vi "MARS_Analysis.vi"() -> ()   [LabVIEW 2015]
uses:
  <vilib>/Analysis/6fits.llb/Curve Fitting Criteria.ctl
  SubVis/MARS_Global_var.vi
  SubVis/Data_Analysis_subvis/MARS_Scan_Data_Analysis_global.vi
  SubVis/Data_Analysis_subvis/ESA_Data_Analysis_Global_VIs.vi
  SubVis/MARS_Scan_Global_var.vi
  <vilib>/Analysis/NI_AALPro.lvlib
panel:
  in  "index":i32=1
  in  "Init std":dbl=1.0 format="%#_13g"
  in  "width":i32=5
  in  "threshold":dbl=10.0 format="%#_13g"
  in  "Discr. Slope":dbl
  in  "Discr. Offset":dbl
  out "Total Counts":i32
  out "Gamma Counts":i32
  out "Neutron Counts":i32
  out "Gamma %":dbl format="%#.2f"
  out "Neutron  %":dbl format="%#.2f"
  in  "Spectrum sel.":bool
  out "Indicator":bool
  in  "Page Selector":enum32{"Free Run Tests", "Scanning Tests"}(radio)
  out "Tab Control":enum32{"Free Run Tests", "Scanning Tests"}(tab)
  in  "Inegral Sel":bool
  in  "Mapping":bool
  in  "Boolean 2":bool
  in  "Spec Selec 2":bool
  out "Spectrum":i32[][](graph)
  out "Int. Graph":i32[][](graph) caption="Intensity Graph"
  out "Scatter":T1(graph) caption="Scatter Plot"
  out "Histogram":i32[][](graph)
  out "FoM":dbl
  out "FoM_1st_min":dbl
  out "FoM_2nd_min":dbl
  out "Channels":i32(listbox) caption="Bckgnd_0.50us-6.00us"
  out "FoM_1st_max":dbl
  out "FoM_2nd_max":dbl
  out "FoM_2":dbl caption="FoM"
  out "Histogram 2":i32[][](graph) caption="Histogram"
  out "Ratio Graph":i32[][](graph) caption="Integral Ratio Graph"
  out "FoM Graph":dbl[][](graph) caption="Optimal FoM"
  in  "Stop Button":bool
  in  "Active Meas.":i32
  out "Meas. Duration (s)":dbl format="%^#.3g"
  out "2nd Integr. (us)":dbl format="%^#.2g"
  out "1st Integr. (us)":dbl format="%^#.2g"
  out "Trigger Level (V)":dbl format="%#.3p"
  in  "Listbox":i32[](listbox) caption="FreeRun_gamma_tests.tdms"
  in  "Read":bool
  out "error out":errorcluster
  # "ADVEOS\nGAEC\nNCSR DEMOKRITOS"
  # "MARS    Neutron Subsystem   Data Analysis"
  # "Neutron-Gamma\nDiscr. Parameters"
  # "Spectrum Statistics"
  # "Measurement Parameters"
  # "%"
  # "%"
  # "Histogram Fit"
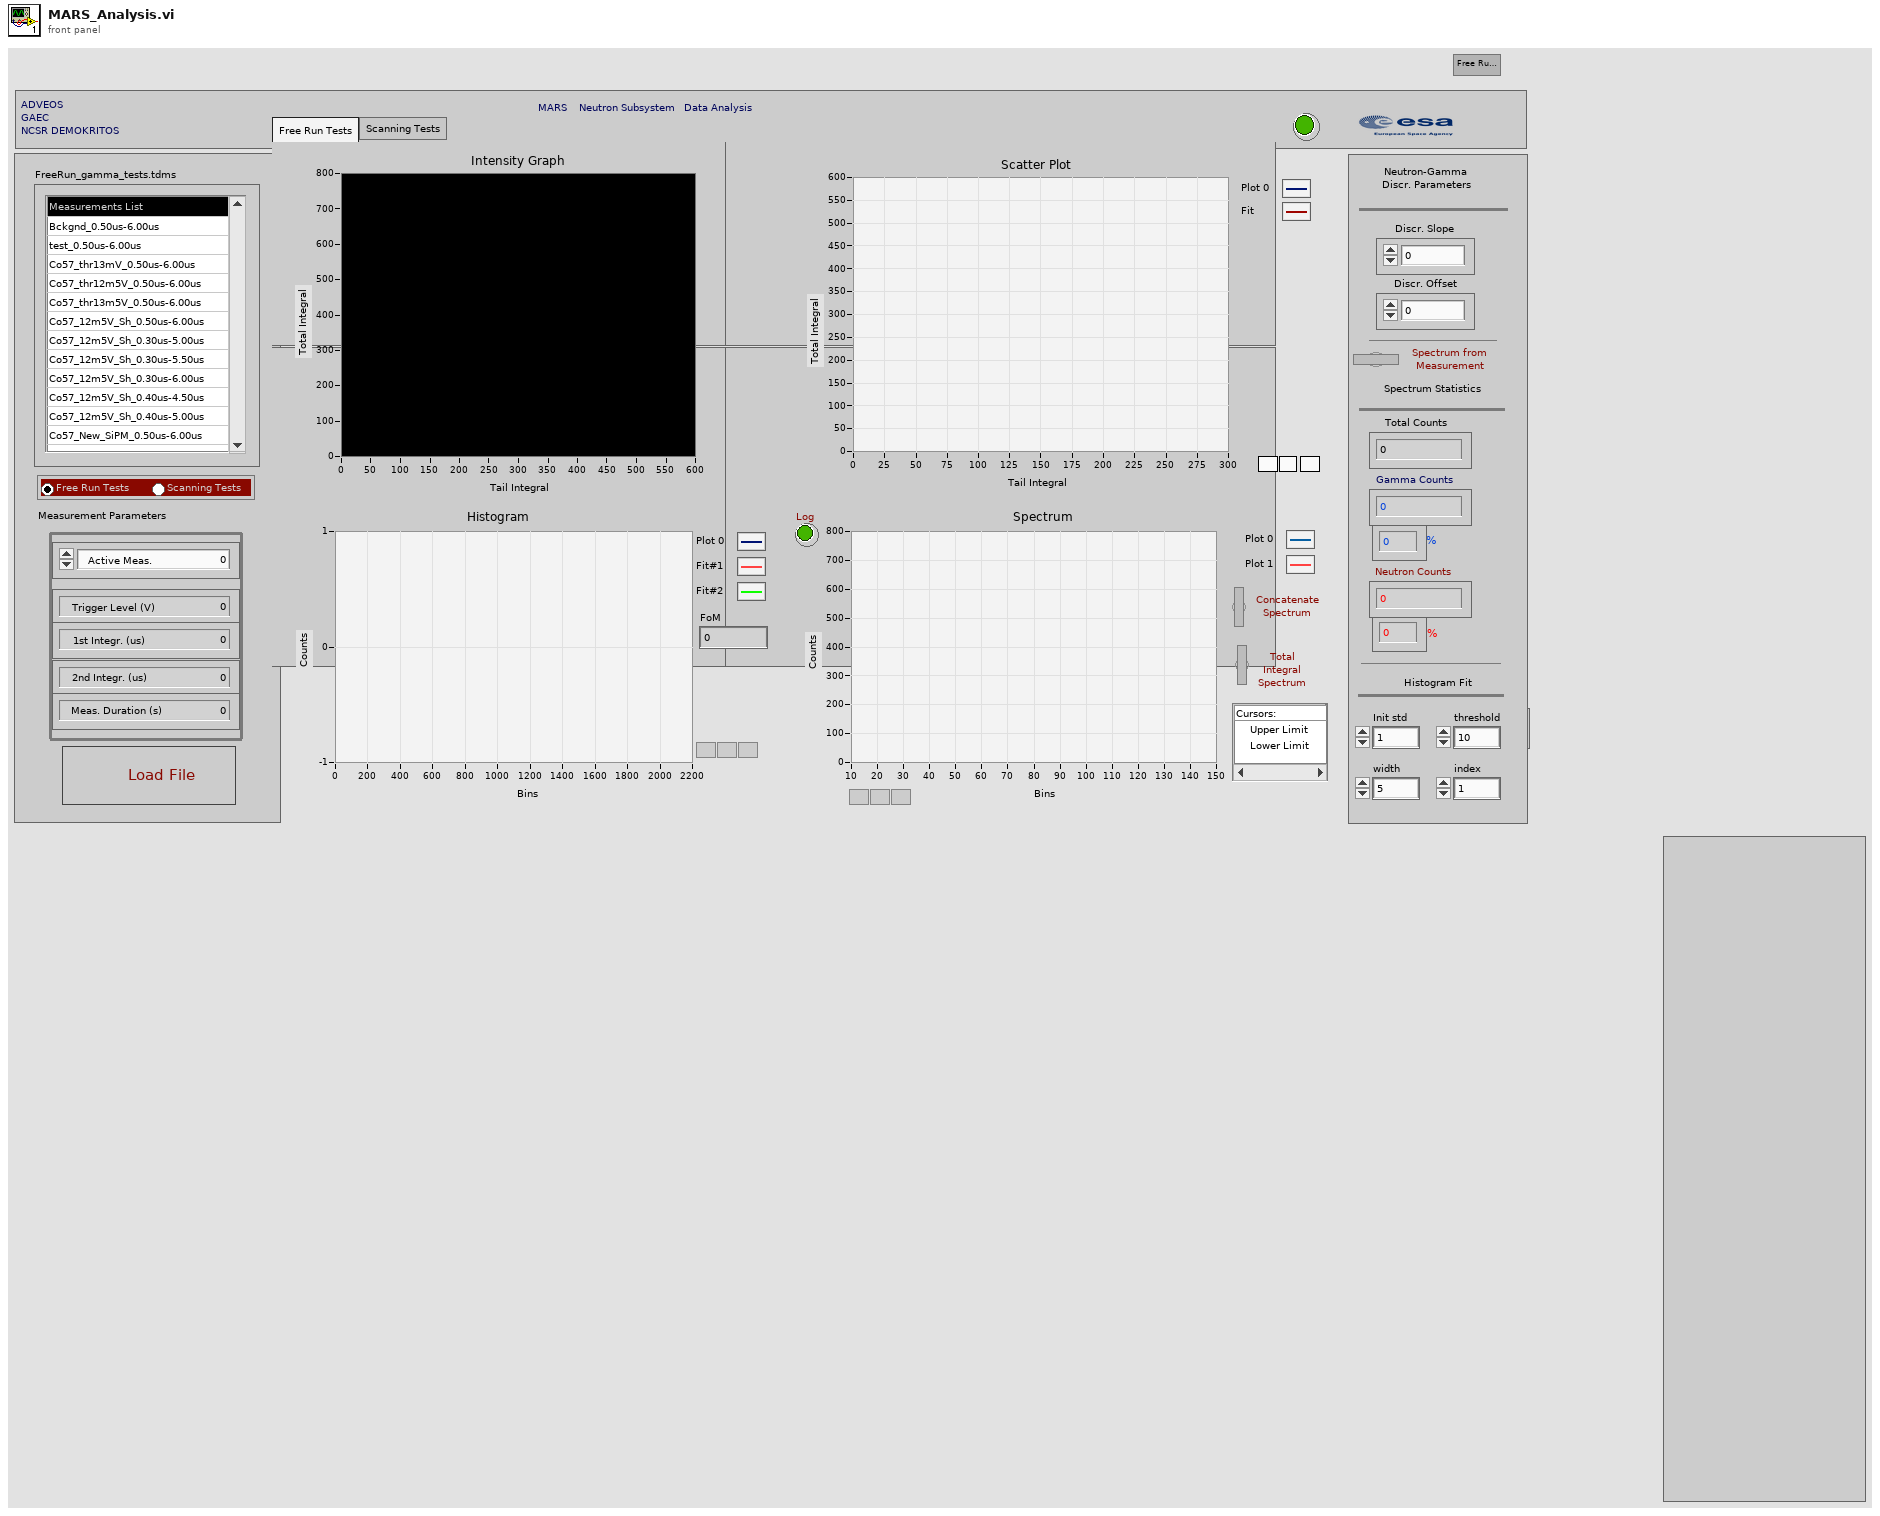
[diagram p1: front panel]
types:
  T1 = cluster{"Tail Integral":i32[], "Total Integral":dbl[]}[]
  T2 = enum16{"open", "open or create", "create or replace", "create", "open (read-only)"}
  T3 = typedef "NI_AALPro.lvlib/Curve Fitting Criteria.ctl" = u16
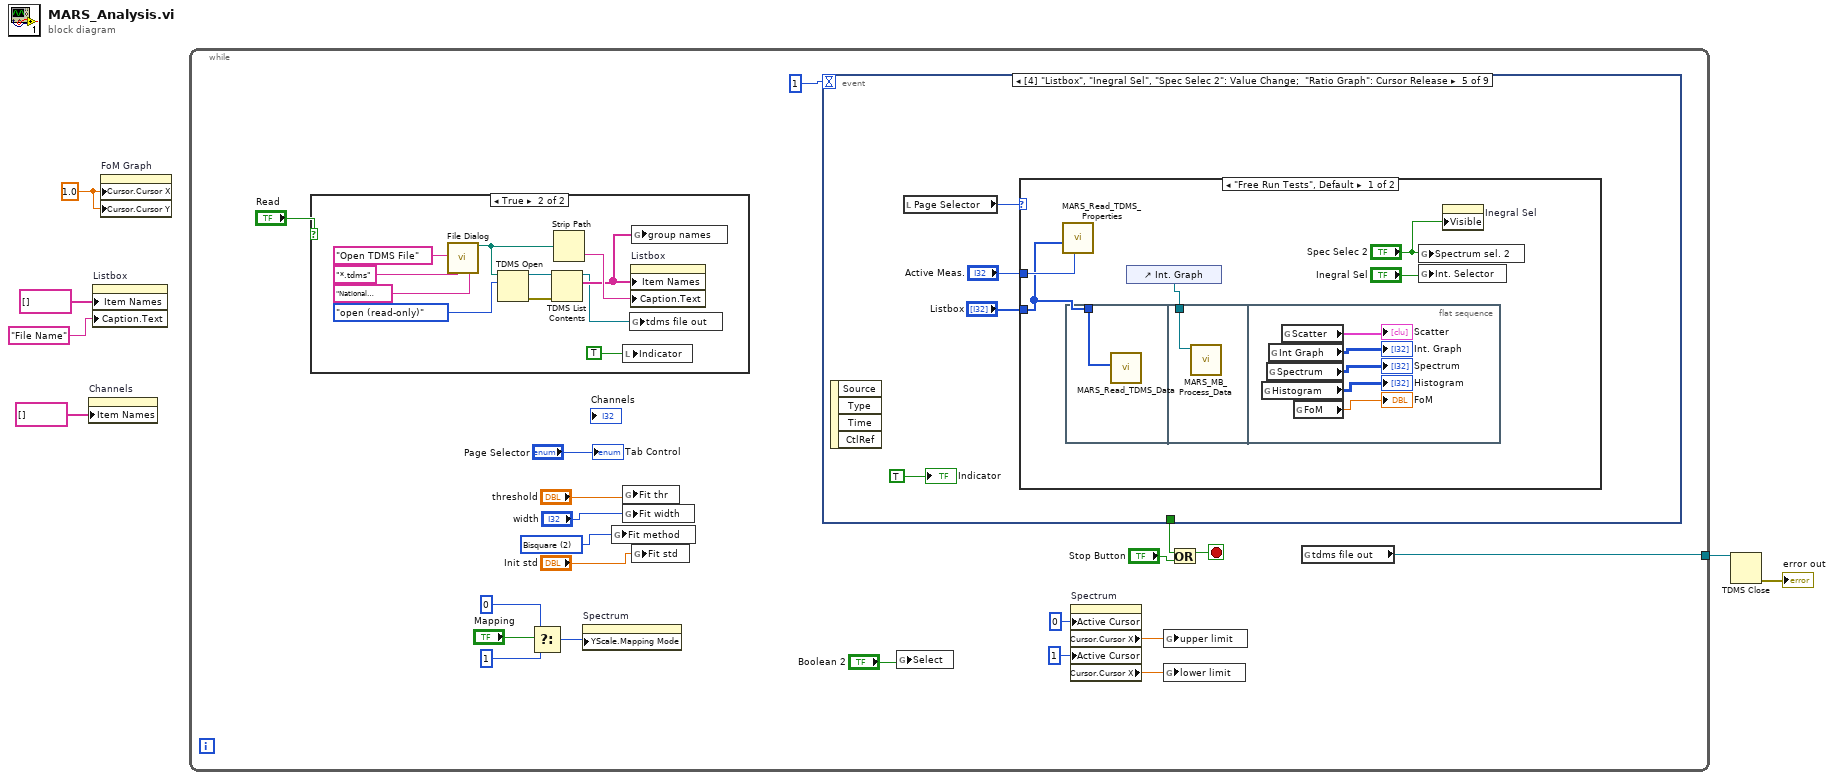
[diagram p0: block diagram]
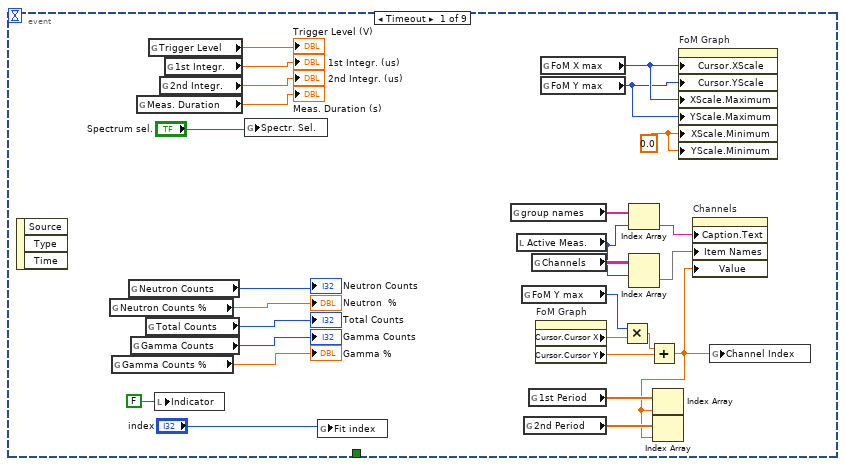
[diagram p3: hidden frame]
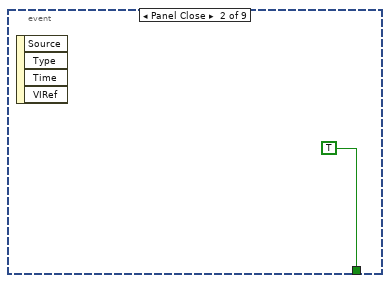
[diagram p4: hidden frame]
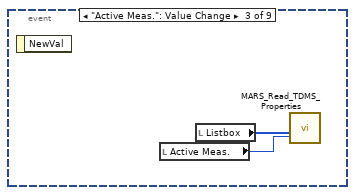
[diagram p5: hidden frame]
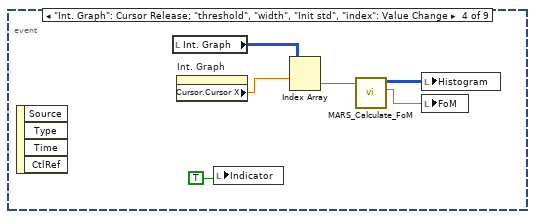
[diagram p6: hidden frame]
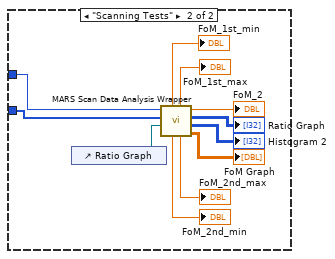
[diagram p7: hidden frame]
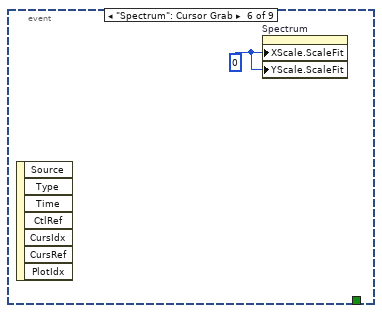
[diagram p8: hidden frame]
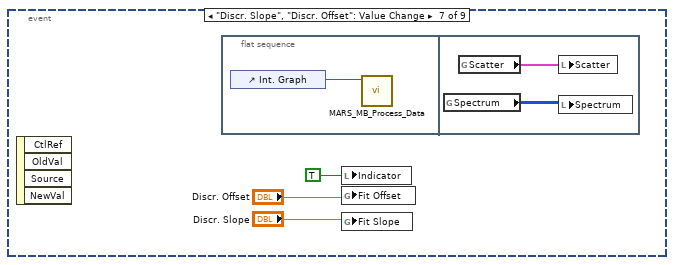
[diagram p9: hidden frame]
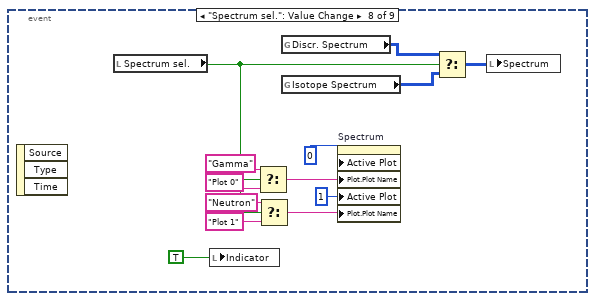
[diagram p10: hidden frame]
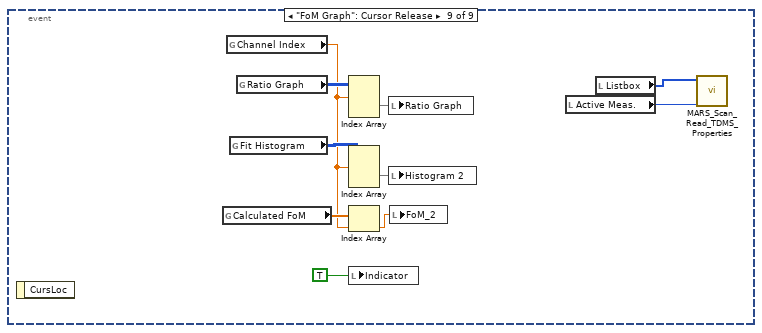
[diagram p11: hidden frame]
diagram:
  w2 = 1.0 ("Cursor.Cursor Position:Cursor X")
  n1 = property on="Channels" class="LstBox (strict)"("Item Names"=string[] []) -> ()  [unwired: 2 in, 2 out]
  n2 = property on="Listbox" class="LstBox (strict)"("Item Names"=string[] [], "Caption.Text"="File Name") -> ()  [unwired: 2 in, 2 out]
  n3 = property on="FoM Graph" class="IntGraph (strict)"("Cursor.Cursor X"=w2, "Cursor.Cursor Y"=w2) -> ()  [unwired: 2 in, 2 out]
  n4 = while {
    tunnel: [w26] -> w6
    stop <- w24 stop-if-true
    w17 = T3 2 items=["Least Square", "Least Absolute Residual", "Bisquare"] ("method")
    n5 = case shown="True" "Read" {
      frame False {
      }
      frame True {
        n6 = call "File Dialog"("prompt"="Open TDMS File" ("prompt tdms"), "pattern (all files)"="*.tdms", "pattern label"="National Instruments TDM Streaming" ("pattern label tdms")) -> ("selected path"=w32:path)  [unwired: 4 in, 8 out]
        n7 = TDMS Open(10:T2."open (read-only)" ("operation (0:open)"), 11:w32) -> (0:w33:errorcluster, 3:w29:refnum<k34>)  [unwired: 5 in]
        n8 = TDMS List Contents(4:w33, 7:w29) -> (2:w30:string[], 3:w28:refnum<k34>)  [unwired: 1 in, 2 out]
        n9 = Strip Path(path=w32) -> (name=w31:string)  [unwired: 1 out]
        n10 = local write "Indicator"(TRUE ("Indicator")) -> ()
        n11 = global write "ESA_Data_Analysis_Global_VIs.vi" "tdms file out"(w28) -> ()
        n12 = property on="Listbox" class="LstBox (strict)"("Item Names"=w30, "Caption.Text"=w31) -> ()  [unwired: 2 in, 2 out]
        n13 = global write "ESA_Data_Analysis_Global_VIs.vi" "group names"(w30) -> ()
      }
    }
    n14 = Select(t=0, s="Mapping", f=1) -> (s? t:f=w9:i32)
    n15 = property on="Spectrum" class="WFGraph (strict)"("YScale.Mapping Mode"=w9) -> ()  [unwired: 2 in, 2 out]
    n16 = global write "MARS_Scan_Global_var.vi" "Fit method"(w17) -> ()
    n17 = global write "MARS_Scan_Global_var.vi" "Fit thr"("threshold") -> ()
    n18 = global write "MARS_Scan_Global_var.vi" "Fit width"("width") -> ()
    n19 = global write "MARS_Scan_Global_var.vi" "Fit std"("Init std") -> ()
    n20 = event shown="[4] \"Listbox\", \"Inegral Sel\", \"Spec Selec 2\": Value Change;  \"Ratio Graph\": Cursor Release" {
      selector: _ -> [_ _ _ _ _ _ _ _ _]
      dyn-events: _ -> [_ _ _ _ _ _ _ _ _]
      timeout: 1 -> [_ _ _ _ _ _ _ _ _]
      tunnel: [_ TRUE ("x") _ _ _ _ _ _ _] -> w22
      event Timeout {
        w40 = 0.0 ("X Scale.Range:Minimum")
        n21 = event-data() -> ()  [unwired: 1 in, 3 out]
        n22 = global read "MARS_Global_var.vi" "Neutron Counts %"() -> (→"Neutron  %":dbl)
        n23 = global read "MARS_Global_var.vi" "Gamma Counts %"() -> (→"Gamma %":dbl)
        n24 = global read "MARS_Global_var.vi" "Neutron Counts"() -> (→"Neutron Counts":i32)
        n25 = global read "MARS_Global_var.vi" "Gamma Counts"() -> (→"Gamma Counts":i32)
        n26 = global read "MARS_Global_var.vi" "Meas. Duration"() -> (→"Meas. Duration (s)":dbl)
        n27 = global read "MARS_Global_var.vi" "Total Counts"() -> (→"Total Counts":i32)
        n28 = global read "MARS_Global_var.vi" "Trigger Level"() -> (→"Trigger Level (V)":dbl)
        n29 = local write "Indicator"(FALSE ("Indicator")) -> ()
        n30 = global read "MARS_Global_var.vi" "2nd Integr."() -> (→"2nd Integr. (us)":dbl)
        n31 = global read "MARS_Global_var.vi" "1st Integr."() -> (→"1st Integr. (us)":dbl)
        n32 = global write "MARS_Global_var.vi" "Spectr. Sel."("Spectrum sel.") -> ()
        n33 = global write "MARS_Global_var.vi" "Fit index"("index") -> ()
        n34 = global read "ESA_Data_Analysis_Global_VIs.vi" "group names"() -> (w49:string[])
        n35 = local read "Active Meas."() -> (w48:i32)
        n36 = global read "MARS_Scan_Data_Analysis_global.vi" "FoM Y max"() -> (w54:i32)
        n37 = global read "MARS_Scan_Data_Analysis_global.vi" "2nd Period"() -> (w51:dbl[])
        n38 = global read "MARS_Scan_Data_Analysis_global.vi" "1st Period"() -> (w52:dbl[])
        n39 = global read "MARS_Scan_Data_Analysis_global.vi" "Channels"() -> (w50:string[][])
        n40 = property on="FoM Graph" class="IntGraph (strict)"() -> ("Cursor.Cursor X"=w53:dbl, "Cursor.Cursor Y"=w56:dbl)  [unwired: 2 in, 2 out]
        n41 = global read "MARS_Scan_Data_Analysis_global.vi" "FoM X max"() -> (w39:i32)
        n42 = global read "MARS_Scan_Data_Analysis_global.vi" "FoM Y max"() -> (w38:i32)
        n43 = Multiply(x=w54, y=w53) -> (x*y=w55:dbl)
        n44 = Index Array(array=w49, index=w48) -> (element=w47:string)
        n45 = Index Array(array=w50, index (row)=w48) -> (element=w46:string[])  [unwired: 1 in]
        n46 = Add(x=w55, y=w56) -> (x+y=w45:dbl)
        n47 = Index Array(array=w52, index=w45) -> ()  [unwired: 1 out]
        n48 = Index Array(array=w51, index=w45) -> ()  [unwired: 1 out]
        n49 = property on="FoM Graph" class="IntGraph (strict)"("Cursor.XScale"=w39, "Cursor.YScale"=w38, "XScale.Maximum"=w39, "YScale.Maximum"=w38, "XScale.Minimum"=w40, "YScale.Minimum"=w40) -> ()  [unwired: 2 in, 2 out]
        n50 = property on="Channels" class="LstBox (strict)"("Caption.Text"=w47, "Item Names"=w46, "Value"=w45) -> ()  [unwired: 2 in, 2 out]
        n51 = global write "MARS_Scan_Data_Analysis_global.vi" "Channel Index"(w45) -> ()
      }
      event Panel Close {
        n52 = event-data() -> ()  [unwired: 1 in, 4 out]
      }
      event "Active Meas.": Value Change {
        n53 = event-data() -> ()  [unwired: 1 in, 1 out]
        n54 = local read "Active Meas."() -> (w66:i32)
        n55 = local read "Listbox"() -> (w67:i32[])
        n56 = call "MARS_Read_TDMS_Properties.vi"("Active Meas."=w66, "Listbox"=w67) -> ()  [unwired: 10 in]
      }
      event "Int. Graph": Cursor Release; "threshold", "width", "Init std", "index": Value Change {
        n57 = event-data() -> ()  [unwired: 1 in, 4 out]
        n58 = local read "Int. Graph"() -> (w73:i32[][])
        n59 = property on="Int. Graph" class="IntGraph (strict)"() -> ("Cursor.Cursor X"=w72:dbl)  [unwired: 2 in, 2 out]
        n60 = local write "Indicator"(TRUE ("Indicator")) -> ()
        n61 = Index Array(array=w73, index (row)=w72) -> (element=w68:i32[])  [unwired: 1 in]
        n62 = call "MARS_Calculate_FoM.vi"("Histogram"=w68) -> ("FoM"=w70:dbl, "Fit Histogram"=w69:i32[][])  [unwired: 9 in]
        n63 = local write "Histogram"(w69) -> ()
        n64 = local write "FoM"(w70) -> ()
      }
      event "Listbox", "Inegral Sel", "Spec Selec 2": Value Change; "Ratio Graph": Cursor Release {
        n65 = event-data() -> ()  [unwired: 1 in, 4 out]
        n66 = local read "Page Selector"() -> (w74:enum32{"Free Run Tests", "Scanning Tests"})
        n67 = case shown="\"Free Run Tests\", Default" w74 {
          tunnel: "Active Meas." -> [w82 w99]
          tunnel: "Listbox" -> [w81 w100]
          frame "Free Run Tests", Default {
            n68 = call "MARS_Read_TDMS_Properties.vi"("Active Meas."=w82, "Listbox"=w81) -> ()  [unwired: 10 in]
            n69 = flat-sequence {
              tunnel: w81 -> [w83]
              tunnel: w80 -> [w84]
              frame #0 {
                n70 = call "MARS_Read_TDMS_Data.vi"("Listbox"=w83) -> ()  [unwired: 11 in]
              }
              frame #1 {
                n71 = call "MARS_MB_Process_Data.vi"("reference"=w84) -> ()  [unwired: 11 in]
              }
              frame #2 {
                n72 = global read "MARS_Global_var.vi" "Histogram"() -> (→"Histogram":i32[][])
                n73 = global read "MARS_Global_var.vi" "Spectrum"() -> (→"Spectrum":i32[][])
                n74 = global read "MARS_Global_var.vi" "Int Graph"() -> (→"Int. Graph":i32[][])
                n75 = global read "MARS_Global_var.vi" "Scatter"() -> (→"Scatter":T1)
                n76 = global read "MARS_Global_var.vi" "FoM"() -> (→"FoM":dbl)
              }
            }
            n77 = control-ref of="Int. Graph"() -> (w80:refnum<vi>)
            n78 = global write "MARS_Global_var.vi" "Spectrum sel. 2"("Spec Selec 2") -> ()
            n79 = global write "MARS_Global_var.vi" "Int. Selector"("Inegral Sel") -> ()
            n80 = property on="Inegral Sel" class="Bool (strict)"("Visible"="Spec Selec 2") -> ()  [unwired: 2 in, 2 out]
          }
          frame "Scanning Tests" {
            n81 = control-ref of="Ratio Graph"() -> (w98:refnum<vi>)
            n82 = call "MARS Scan Data Analysis Wrapper.vi"("Ratio Graph in"=w98, "Listbox"=w100, "Active Meas."=w99) -> ("FoM Graph"=→"FoM Graph":dbl[][], "Fit Histogram"=→"Histogram 2":i32[][], "Ratio Graph"=→"Ratio Graph":i32[][], "FoM"=→"FoM_2":dbl, "FoM_2nd_max"=→"FoM_2nd_max":dbl, "FoM_1st_max"=→"FoM_1st_max":dbl, "FoM_2nd_min"=→"FoM_2nd_min":dbl, "FoM_1st_min"=→"FoM_1st_min":dbl)  [unwired: 1 in]
          }
        }
        "Indicator" <- TRUE ("Indicator")
      }
      event "Spectrum": Cursor Grab {
        w101 = u8 0 ("X Scale.Scale Fit")
        n83 = event-data() -> ()  [unwired: 1 in, 7 out]
        n84 = property on="Spectrum" class="WFGraph (strict)"("XScale.ScaleFit"=w101, "YScale.ScaleFit"=w101) -> ()  [unwired: 2 in, 2 out]
      }
      event "Discr. Slope", "Discr. Offset": Value Change {
        n85 = event-data() -> ()  [unwired: 1 in, 4 out]
        n86 = flat-sequence {
          frame #0 {
            n87 = control-ref of="Int. Graph"() -> (w105:refnum<vi>)
            n88 = call "MARS_MB_Process_Data.vi"("reference"=w105) -> ()  [unwired: 11 in]
          }
          frame #1 {
            n89 = global read "MARS_Global_var.vi" "Spectrum"() -> (w107:i32[][])
            n90 = global read "MARS_Global_var.vi" "Scatter"() -> (w106:T1)
            n91 = local write "Scatter"(w106) -> ()
            n92 = local write "Spectrum"(w107) -> ()
          }
        }
        n93 = local write "Indicator"(TRUE ("Indicator")) -> ()
        n94 = global write "MARS_Global_var.vi" "Fit Offset"("Discr. Offset") -> ()
        n95 = global write "MARS_Global_var.vi" "Fit Slope"("Discr. Slope") -> ()
      }
      event "Spectrum sel.": Value Change {
        n96 = event-data() -> ()  [unwired: 1 in, 3 out]
        n97 = local read "Spectrum sel."() -> (w110:bool)
        n98 = local write "Indicator"(TRUE ("Indicator")) -> ()
        n99 = Select(t="Gamma" ("Plot.Plot Name"), s=w110, f="Plot 0") -> (s? t:f=w120:string)
        n100 = Select(t="Neutron" ("Plot.Plot Name"), s=w110, f="Plot 1") -> (s? t:f=w116:string)
        n101 = global read "MARS_Global_var.vi" "Discr. Spectrum"() -> (w112:i32[][])
        n102 = global read "MARS_Global_var.vi" "Isotope Spectrum"() -> (w111:i32[][])
        n103 = property on="Spectrum" class="WFGraph (strict)"("Active Plot"=u32 0, "Plot.Plot Name"=w120, "Active Plot"=u32 1, "Plot.Plot Name"=w116) -> ()  [unwired: 2 in, 2 out]
        n104 = Select(t=w112, s=w110, f=w111) -> (s? t:f=w108:i32[][])
        n105 = local write "Spectrum"(w108) -> ()
      }
      event "FoM Graph": Cursor Release {
        n106 = event-data() -> ()  [unwired: 1 in, 1 out]
        n107 = global read "MARS_Scan_Data_Analysis_global.vi" "Calculated FoM"() -> (w126:dbl[])
        n108 = global read "MARS_Scan_Data_Analysis_global.vi" "Channel Index"() -> (w125:dbl)
        n109 = global read "MARS_Scan_Data_Analysis_global.vi" "Fit Histogram"() -> (w129:i32[][][])
        n110 = global read "MARS_Scan_Data_Analysis_global.vi" "Ratio Graph"() -> (w130:i32[][][])
        n111 = Index Array(array=w130, index (dim 0)=w125) -> (element=w128:i32[][])  [unwired: 2 in]
        n112 = Index Array(array=w129, index (dim 0)=w125) -> (element=w127:i32[][])  [unwired: 2 in]
        n113 = Index Array(array=w126, index=w125) -> (element=w124:dbl)
        n114 = local write "Indicator"(TRUE ("Indicator")) -> ()
        n115 = local write "Ratio Graph"(w128) -> ()
        n116 = local write "Histogram 2"(w127) -> ()
        n117 = local write "FoM_2"(w124) -> ()
        n118 = local read "Active Meas."() -> (w121:i32)
        n119 = local read "Listbox"() -> (w122:i32[])
        n120 = call "MARS_Scan_Read_TDMS_Properties.vi"("Active Meas."=w121, "Listbox"=w122) -> ()  [unwired: 10 in]
      }
    }
    n121 = global write "MARS_Global_var.vi" "Select"("Boolean 2") -> ()
    n122 = property on="Spectrum" class="WFGraph (strict)"("Active Cursor"=u32 0, "Active Cursor"=u32 1) -> ("Cursor.Cursor X"=w12:dbl, "Cursor.Cursor X"=w13:dbl)  [unwired: 2 in, 2 out]
    n123 = global write "MARS_Global_var.vi" "upper limit"(w12) -> ()
    n124 = global write "MARS_Global_var.vi" "lower limit"(w13) -> ()
    n125 = Or(x=w22, y="Stop Button") -> (x .or. y?=w24:bool)
    n126 = global read "ESA_Data_Analysis_Global_VIs.vi" "tdms file out"() -> (w26:refnum<k34>)
    "Tab Control" <- "Page Selector"
  }
  n127 = TDMS Close(11:w6) -> (0:→"error out":errorcluster)  [unwired: 1 in, 1 out]
